vi "store_plot.vi"(6 "Reset? (F)":bool, 10 "Ch to Sample":bool[](array[boolean]), 11 "Output Plot":cluster{"X2":dbl[], "Y2":dbl[]}[](array[cluster])) -> (2 "Ch to Sample Variable":bool[][](array[boolean]), 3 "Plot Variable":cluster{"X2":dbl[], "Y2":dbl[]}[][](array[cluster]))   [LabVIEW 2020]
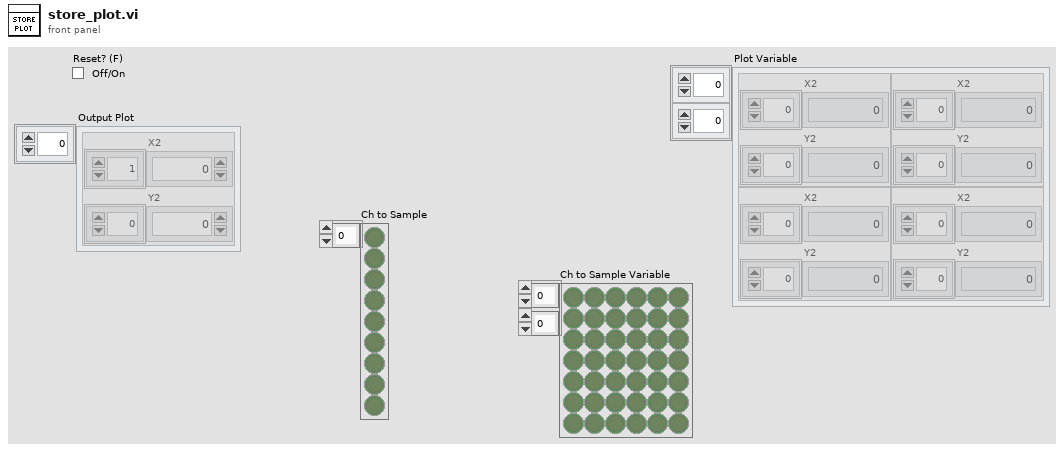
[diagram p1: front panel]
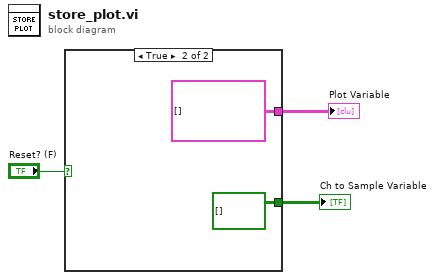
[diagram p0: block diagram]
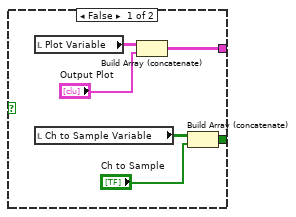
[diagram p2: hidden frame]
diagram:
  n1 = case shown="True" "Reset? (F)" {
    tunnel: [w7 bool[][] []] -> w3
    tunnel: [w4 cluster{"X2":dbl[], "Y2":dbl[]}[][] []] -> w2
    frame False {
      n2 = local read "Plot Variable"() -> (w6:cluster{"X2":dbl[], "Y2":dbl[]}[][])
      n3 = local read "Ch to Sample Variable"() -> (w5:bool[][])
      n4 = Build Array (concatenate)(w6, "Output Plot") -> (w4:cluster{"X2":dbl[], "Y2":dbl[]}[][])
      n5 = Build Array (concatenate)(w5, "Ch to Sample") -> (w7:bool[][])
    }
    frame True {
    }
  }
  "Plot Variable" <- w2
  "Ch to Sample Variable" <- w3
